vi "SemiActiveScheduler.vi"(8 "Proocessing Times":i32[](array[numeric]), 9 "Schedule":i32[](array[numeric]), 10 "Number Of Machines":i32, 11 "Number Of Jobs":i32) -> (1 "EOJ":i32[](array[numeric]), 2 "EOM":i32[](array[numeric]), 3 "Job Completion Times":i32[](array[numeric]))   [LabVIEW 2013]
uses:
  Classes/Scheduler.lvclass
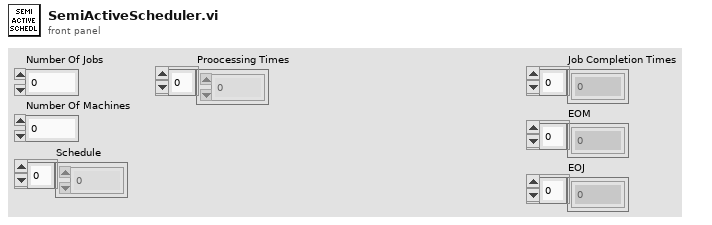
[diagram p1: front panel]
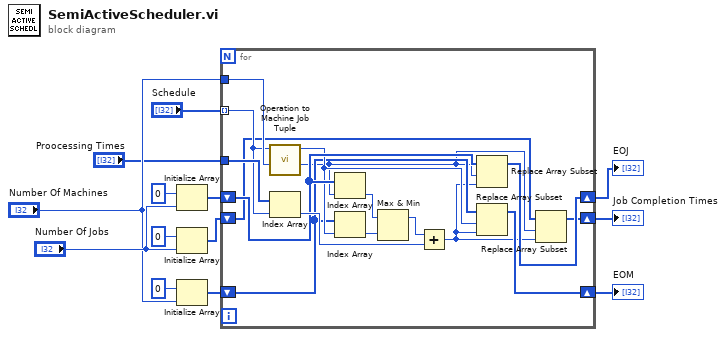
[diagram p0: block diagram]
diagram:
  n1 = Initialize Array(0, "Number Of Jobs") -> (w7:i32[])
  n2 = Initialize Array(0, "Number Of Jobs") -> (w4:i32[])
  n3 = Initialize Array(0, "Number Of Machines") -> (w6:i32[])
  n4 = for {
    tunnel: "Schedule" -> [w25] mode=indexing
    tunnel: "Number Of Machines" -> [w29]
    shift-right: [w21] -> w1
    shift-left: w7 -> [w22]
    shift-right: [w18] -> w2
    shift-left: w6 -> [w19]
    tunnel: "Proocessing Times" -> [w26]
    shift-right: [w14] -> w3
    shift-left: w4 -> [w17]
    n5 = call "Operation to Machine Job Tuple.vi"("Number of Machines"=w29, "Operation Number"=w25) -> ("Job No"=w16:i32, "Machine No"=w20:i32)  [unwired: 8 in]
    n6 = Index Array(array=w26, index=w25) -> (element=w23:i32)
    n7 = Index Array(array=w22, index=w16) -> (element=w28:i32)
    n8 = Index Array(array=w19, index=w20) -> (element=w27:i32)
    n9 = Max & Min(x=w28, y=w27) -> (max(x,y)=w24:i32)  [unwired: 1 out]
    n10 = Add(x=w24, y=w23) -> (x+y=w15:i32)
    n11 = Replace Array Subset(array=w22, new element=w15, index=w16) -> (w21:i32[])
    n12 = Replace Array Subset(array=w19, new element=w15, index=w20) -> (w18:i32[])
    n13 = Replace Array Subset(array=w17, new element=w15, index=w16) -> (w14:i32[])
  }
  "Job Completion Times" <- w3
  "EOM" <- w2
  "EOJ" <- w1
